vi "Update Indicators (Data String to ref array).vi"(1 "Array":refnum<vi>[](array[refnum]), 2 "Active Channel":string, 7 "Data String":string, 11 "error in (no error)":errorcluster) -> (4 "name/data":string[][](array[string]), 15 "error out":errorcluster)   [LabVIEW 2020]
panel:
  out "Array 5":string[](array[string])
  out "subarray":string[](array[string])
  out "Array 4":string[][](array[string])
  out "Array 2":string[](array[string])
  out "Array 3":string[](array[string])
  out "Label.Text 3":string
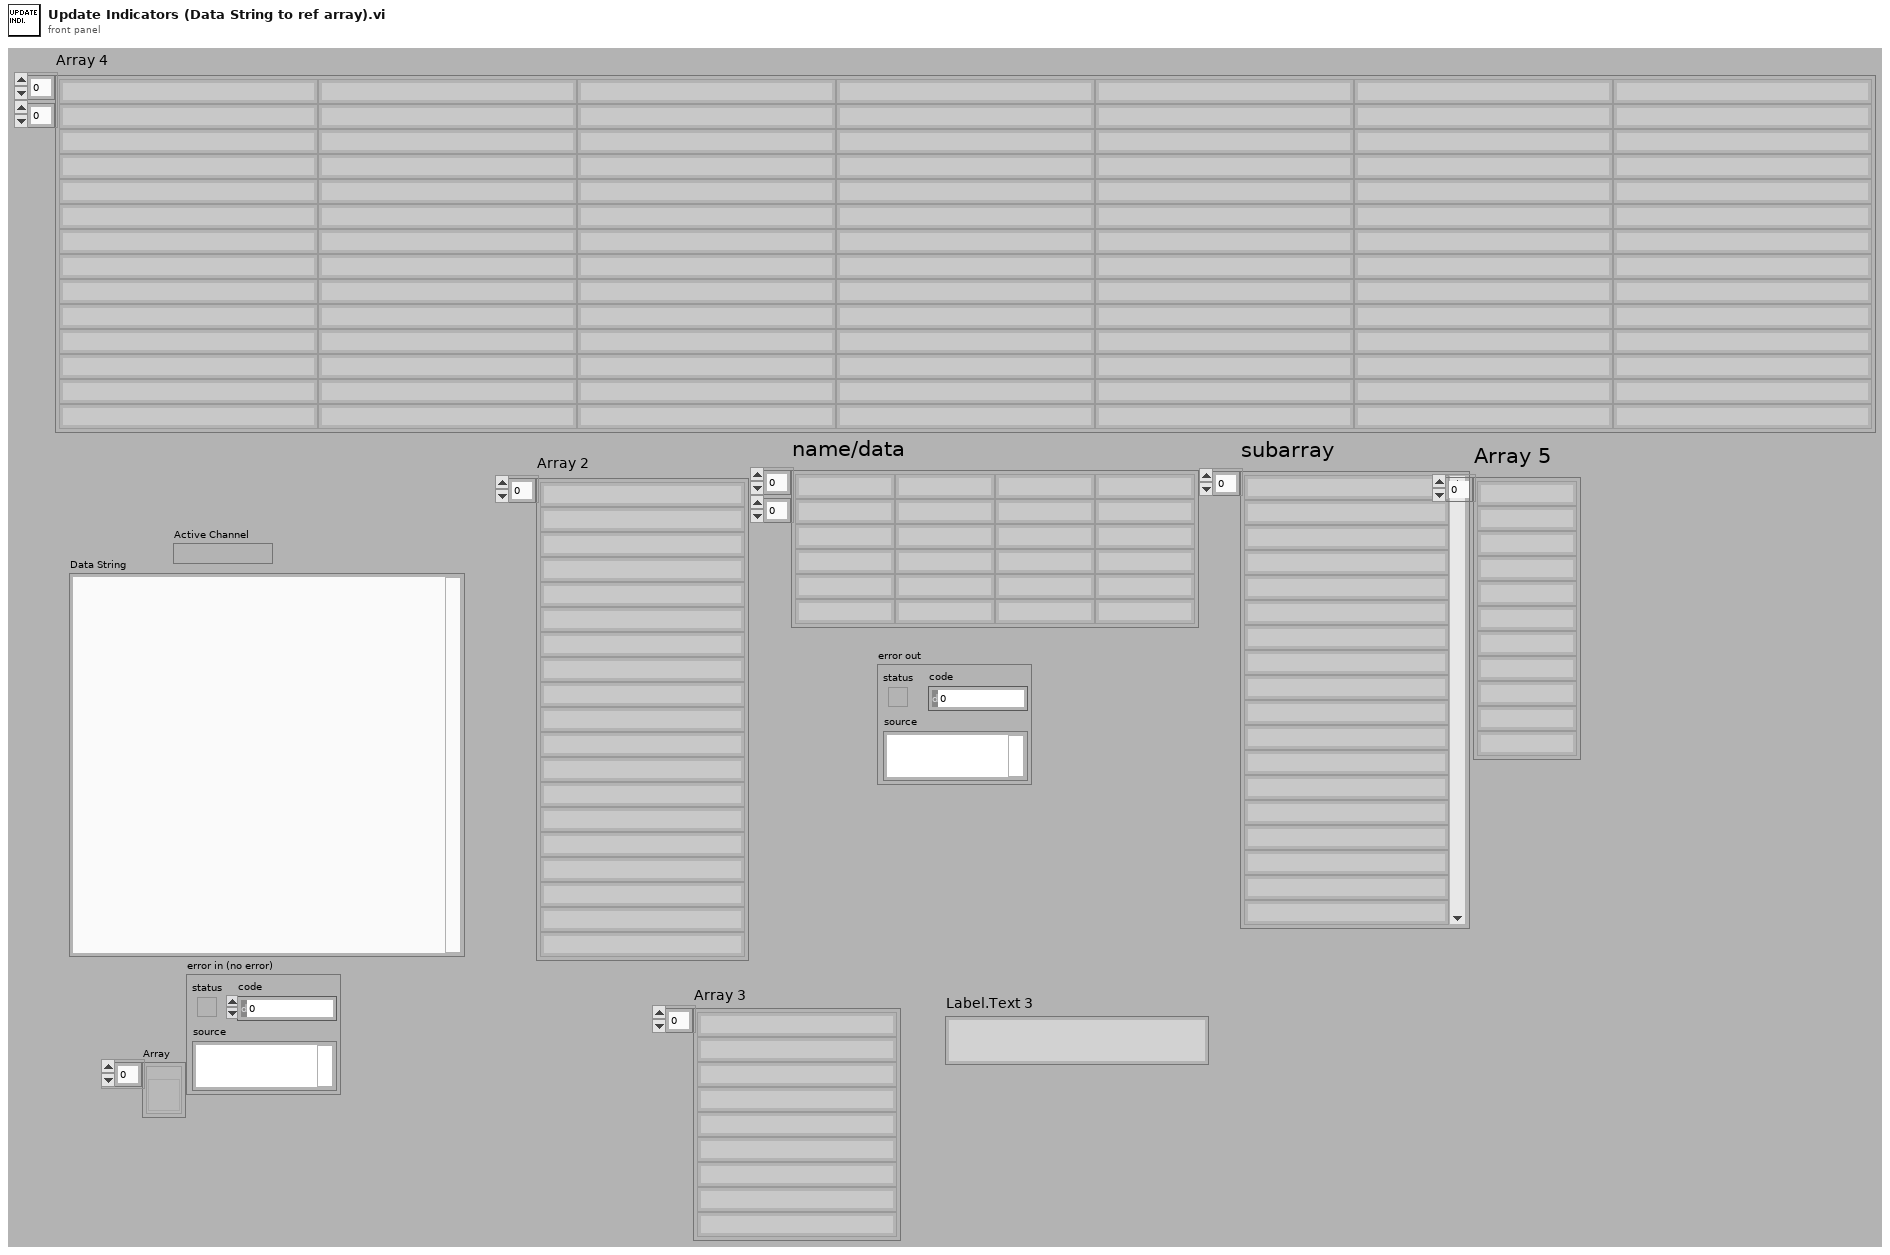
[diagram p1: front panel]
types:
  T1 = typedef "Type Descriptor Enumeration__ogtk.ctl" = enum8{"<Null>", "I8", "I16", "I32", "I64", "U8", "U16", "U32", "U64", "SGL", "DBL", "EXT", "CSG", "CDB", "CXT", "0x0F", "0x10", "0x11", "0x12", "0x13", "0x14", "Enum U8", "Enum U16", "Enum U32", "Enum U64", "SGL PQ", "DBL PQ", "EXT PQ", "CSG PQ", "CDB PQ", "CXT PQ", "0x1F", "0x20", "Boolean", "0x22", "0x23", "0x24", "0x25", "0x26", "0x27", "0x28", "0x29", "0x2A", "0x2B", "0x2C", "0x2D", "0x2E", "0x2F", "String", "0x31", "Path", "Pict", "0x34", "0x35", "0x36", "DAQ", "0x38", "0x39", "0x3A", "0x3B", "0x3C", "0x3D", "0x3E", "0x3F", "Array", "0x41", "0x42", "0x43", "0x44", "0x45", "0x46", "0x47", "0x48", "0x49", "0x4A", "0x4B", "0x4C", "0x4D", "0x4E", "0x4F", "Cluster", "0x51", "0x52", "Variant", "Waveform", "0x55", "0x56", "0x57", "0x58", "0x59", "0x5A", "0x5B", "0x5C", "0x5D", "0x5E", "0x5F", "0x60", "0x61", "0x62", "0x63", "0x64", "0x65", "0x66", "0x67", "0x68", "0x69", "0x6A", "0x6B", "0x6C", "0x6D", "0x6E", "0x6F", "Refnum"}
  T2 = enum8{"Enabled", "Disabled", "Disabled and Grayed Out"}
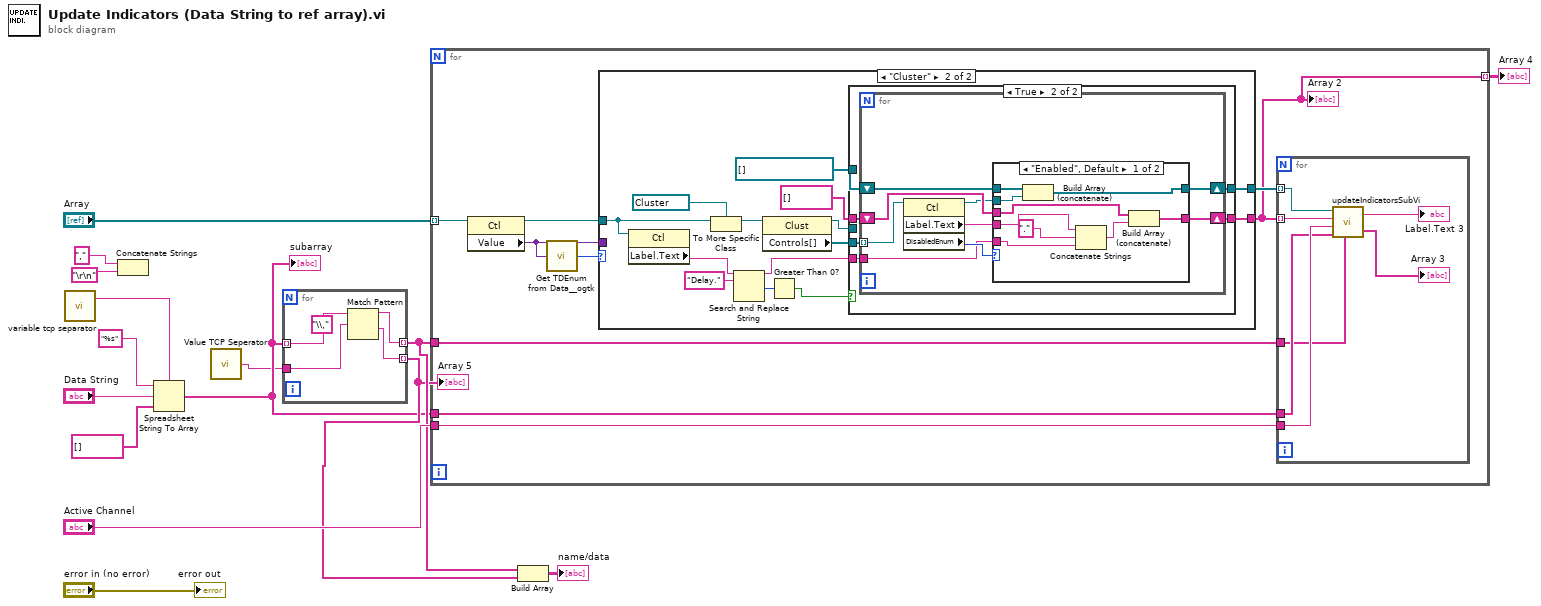
[diagram p0: block diagram]
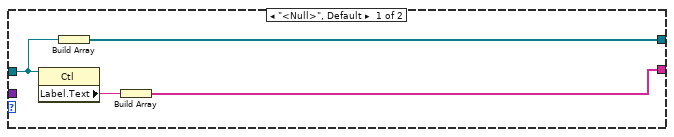
[diagram p2: hidden frame]
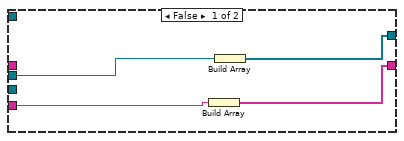
[diagram p3: hidden frame]
diagram:
  n1 = call "variable tcp separator.vi"() -> ("variable separator"=w2:string)  [unwired: 3 in]
  n2 = Concatenate Strings("," ("string"), "\r\n") -> ()  [unwired: 1 out]
  n3 = Spreadsheet String To Array(delimiter (Tab)=w2, format string="%s", spreadsheet string="Data String", array type (2D Dbl)=string[] []) -> (array=w3:string[])
  "subarray" <- w3
  n4 = call "Value TCP Seperator.vi"() -> ("Value TCP Seperator"=w1:string)  [unwired: 1 in]
  n5 = for {
    tunnel: w3 -> [w19] mode=indexing
    tunnel: [w18] -> w9 mode=indexing
    tunnel: [w17] -> w8 mode=indexing
    tunnel: w1 -> [w16]
    (unwired) "\\," ("regular expression")
    n6 = Match Pattern(string=w19, regular expression=w16) -> (before substring=w18:string, after substring=w17:string)  [unwired: 1 in, 2 out]
  }
  "Array 5" <- w8
  n7 = for {
    tunnel: "Array" -> [w25] mode=indexing
    tunnel: w9 -> [w26]
    tunnel: "Active Channel" -> [w28]
    tunnel: w3 -> [w27]
    tunnel: [w20] -> w10 mode=indexing
    n8 = property class="Ctl"(reference=w25) -> (reference out=w22:refnum<vi>, "Value"=w23:variant)  [unwired: 1 in, 1 out]
    n9 = call <userlib>:"Get TDEnum from Data__ogtk.vi"("Data"=w23) -> ("Type Descriptor Enumeration"=w24:T1)  [unwired: 4 in]
    n10 = case shown="\"Cluster\"" w24 {
      tunnel: w23 -> [_ _]
      tunnel: w22 -> [w38 w46]
      tunnel: [w36 w50] -> w20
      tunnel: [w39 w48] -> w21
      frame "<Null>", Default {
        n11 = property class="Ctl"(reference=w38) -> ("Label.Text"=w37:string)  [unwired: 1 in, 2 out]
        n12 = Build Array(w38) -> (w39:refnum<vi>[])
        n13 = Build Array(w37) -> (w36:string[])
      }
      frame "Cluster" {
        n14 = property class="Ctl"(reference=w46) -> ("Label.Text"=w45:string)  [unwired: 1 in, 2 out]
        n15 = To More Specific Class(target class=refnum<vi> refnum ("specific class reference"), reference=w46) -> (specific class reference=w52:refnum<vi>)  [unwired: 1 in, 1 out]
        n16 = Search and Replace String(input string=w45, search string="Delay.") -> (result string=w44:string, number of replacements=w42:i32)  [unwired: 6 in, 2 out]
        n17 = property class="Clust"(reference=w52) -> (reference out=w40:refnum<vi>, "Controls[]"=w51:refnum<vi>[])  [unwired: 1 in, 1 out]
        n18 = Greater Than 0?(x=w42) -> (x > 0?=w41:bool)
        n19 = case shown="True" w41 {
          tunnel: w51 -> [_ w63]
          tunnel: [w56 w62] -> w50
          tunnel: refnum<vi>[] [] -> [_ w61]
          tunnel: [w54 w60] -> w48
          tunnel: string[] [] -> [_ w59]
          tunnel: w44 -> [w57 w58]
          tunnel: w40 -> [w55 _]
          frame False {
            n20 = Build Array(w57) -> (w56:string[])
            n21 = Build Array(w55) -> (w54:refnum<vi>[])
          }
          frame True {
            n22 = for {
              tunnel: w63 -> [w72] mode=indexing
              shift-right: [w69] -> w62
              shift-left: w59 -> [w71]
              shift-right: [w66] -> w60
              shift-left: w61 -> [w65]
              tunnel: w58 -> [w64]
              n23 = property class="Ctl"(reference=w72) -> (reference out=w67:refnum<vi>, "Label.Text"=w70:string, "DisabledEnum"=w68:T2)  [unwired: 1 in, 1 out]
              n24 = case shown="\"Enabled\", Default" w68 {
                tunnel: w71 -> [w80 w83]
                tunnel: w70 -> [w74 _]
                tunnel: [w81 w83] -> w69
                tunnel: w67 -> [w79 _]
                tunnel: [w78 w82] -> w66
                tunnel: w65 -> [w77 w82]
                tunnel: w64 -> [w75 _]
                frame "Enabled", Default {
                  n25 = Build Array (concatenate)(w77, w79) -> (w78:refnum<vi>[])
                  n26 = Concatenate Strings(w74, "." ("string"), w75) -> (w73:string)
                  n27 = Build Array (concatenate)(w80, w73) -> (w81:string[])
                }
                frame "Disabled" {
                }
              }
            }
          }
        }
      }
    }
    "Array 2" <- w20
    n28 = for {
      tunnel: w28 -> [w35]
      tunnel: w21 -> [w34] mode=indexing
      tunnel: w27 -> [w33]
      tunnel: w26 -> [w32]
      tunnel: w20 -> [w31] mode=indexing
      n29 = call "updateIndicatorsSubVi.vi"("trigger"=w34, "Label.Text"=w31, "Active Channel"=w35, "Array 2"=w33, "Array"=w32) -> ("Label.Text 3"=→"Label.Text 3":string, "Array 3"=→"Array 3":string[])
    }
  }
  "Array 4" <- w10
  n30 = Build Array(w9, w8) -> (→"name/data":string[][])
  "error out" <- "error in (no error)"
